vi "Read Port.vi"(8 "error in (no error)":errorcluster, 9 "Timeout":i16, 11 "MPU in":refnum<class "MPU.lvclass">) -> (0 "error out":errorcluster, 1 "Timeouted":bool, 2 "Data":u8, 3 "MPU out":refnum<class "MPU.lvclass">)   [LabVIEW 2018, in "Modbus_Processing_Unit.lvlib" / "MPU.lvclass"]
uses:
  MPU.lvclass
  MPU.lvclass/MPU.ctl
  <vilib>/rvi/eio/common/nirviEmuTemplateMethod_errors.vi
  <vilib>/eio/EIOMethodNode/EIOMethodNode.xnode
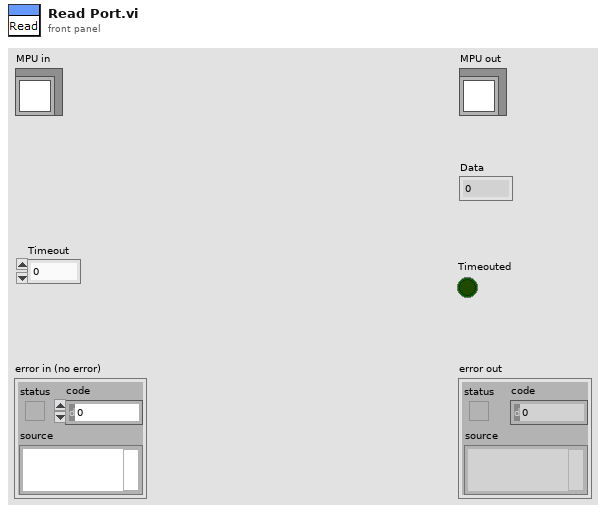
[diagram p1: front panel]
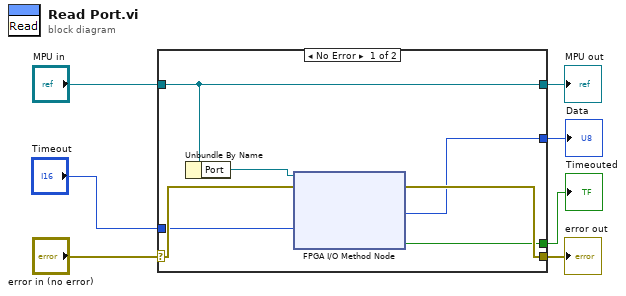
[diagram p0: block diagram]
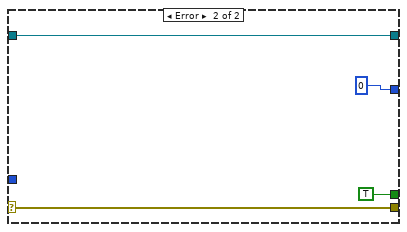
[diagram p2: hidden frame]
diagram:
  n1 = case shown="No Error" "error in (no error)" {
    selector: "error in (no error)" -> [w12 w17]
    tunnel: [w11 w17] -> w6
    tunnel: [w14 w18] -> w4
    tunnel: "MPU in" -> [w14 w18]
    tunnel: "Timeout" -> [w10 _]
    tunnel: [w9 u8 0 ("Data")] -> w1
    tunnel: [w8 TRUE ("Timed Out")] -> w2
    frame No Error {
      n2 = Unbundle By Name(w14) -> ("Port"=w13:refnum<k21>)
      n3 = xnode "FPGA I/O Method Node"("error in"=w12, "FPGA I/O In"=w13, "Timeout (ms)"=w10) -> ("error out"=w11:errorcluster, "Data"=w9:u8, "Timed Out"=w8:bool)  [unwired: 1 out]
    }
    frame Error {
    }
  }
  "error out" <- w6
  "MPU out" <- w4
  "Data" <- w1
  "Timeouted" <- w2
